vi "ATF Storage-Data to host.vi"(8 "error in (no error)":errorcluster, 11 "Err":refnum<queue>) -> (0 "error out":errorcluster, 3 "Data":string)   [LabVIEW 2022 SP3]
uses:
  RT Controls/ATF Storage-Data Type Control screen.ctl
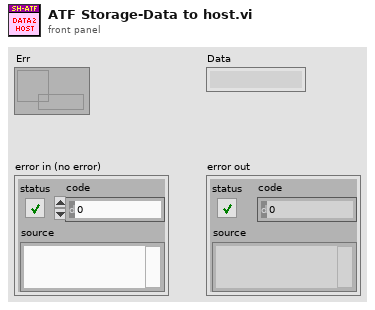
[diagram p1: front panel]
types:
  T1 = typedef "ATF Storage-Data Type Control screen.ctl" = cluster{"DI_Data":digitalwaveform[], "Drive_A_C":waveform(dbl)[], "Drive_A_D":waveform(dbl)[], "Drive_L_C":waveform(dbl)[], "Drive_L_D":waveform(dbl)[], "Loop Status":bool[], "CDT Timer":dbl, "RT Error":cluster{"Error Code":string, "Error Source":string}, "DO":waveform(dbl)[], "SEQ Monitor":string[], "Device List":string}
  T2 = enum16{"Init", "Read 'All'", "Read 'n'", "Read '1'", "Write '1'", "Write 'n'", "Write 'All'"}
  T3 = cluster{"Error Code":string, "Error Source":string}
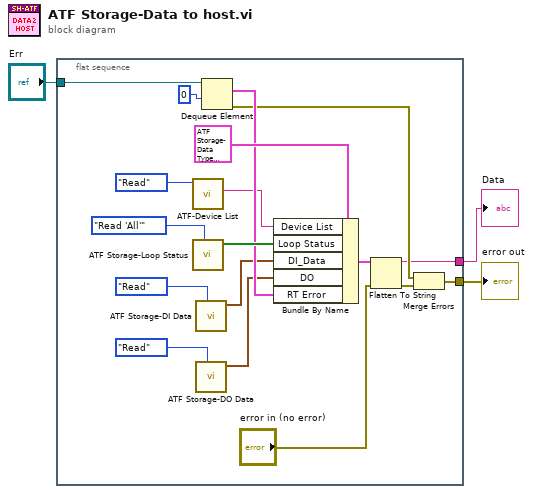
[diagram p0: block diagram]
diagram:
  n1 = flat-sequence {
    tunnel: "Err" -> [w21]
    tunnel: [w5] -> w2
    tunnel: [w4] -> w1
    frame #0 {
      n2 = call "ATF-Device List.vi"("Enum"=enum16{"Write", "Read"}."Read") -> ("DL 2"=w10:string)  [unwired: 9 in, 1 out]
      n3 = call "ATF Storage-Loop Status.vi"("Option"=T2."Read 'All'") -> ("Status List Out"=w19:bool[])  [unwired: 8 in, 2 out]
      n4 = call "ATF Storage-DI Data.vi"("Enum"=enum16{"Write", "Read"}."Read") -> ("Out_DI data"=w14:digitalwaveform[])  [unwired: 10 in]
      n5 = call "ATF Storage-DO Data.vi"("Enum"=enum16{"Write", "Read"}."Read") -> ("out_DO data"=w12:waveform(dbl)[])  [unwired: 10 in]
      n6 = Dequeue Element(queue=w21, timeout in ms (-1)=0) -> (element=w16:T3, error out=w7:errorcluster)  [unwired: 1 in, 2 out]
      n7 = Bundle By Name(cluster=T1 {"DI_Data"=[], "Drive_A_C"=[], "Drive_A_D"=[], "Drive_L_C"=[], "Drive_L_D"=[], "Loop Status"=[], "CDT Timer"=0.0, "RT Error"={"Error Code"="", "Error Source"=""}, "DO"=[], "SEQ Monitor"=[], "Device List"=""} ("Cluster"), "Device List"=w10, "Loop Status"=w19, "DI_Data"=w14, "DO"=w12, "RT Error"=w16) -> (w9:T1)
      n8 = Flatten To String(anything=w9, error in (no error)="error in (no error)") -> (data string=w4:string, error out=w6:errorcluster)  [unwired: 2 in, 1 out]
      n9 = Merge Errors(w7, w6) -> (w5:errorcluster)
    }
  }
  "error out" <- w2
  "Data" <- w1
